vi "blink_if_zero.vi"(8 "error in (no error)":errorcluster, 11 "ImagingModeDL100901FlexTrajectory in":refnum<class "ImagingModeDL100901FlexTrajectory.lvclass">) -> (0 "error out":errorcluster, 3 "ImagingModeDL100901FlexTrajectory out":refnum<class "ImagingModeDL100901FlexTrajectory.lvclass">)   [LabVIEW 2010, in "ImagingModeDL100901FlexTrajectory.lvclass"]
uses:
  ImagingModeDL100901FlexTrajectory.lvclass
  ImagingModeDL100901FlexTrajectory.lvclass/ImagingModeDL100901FlexTrajectory.ctl
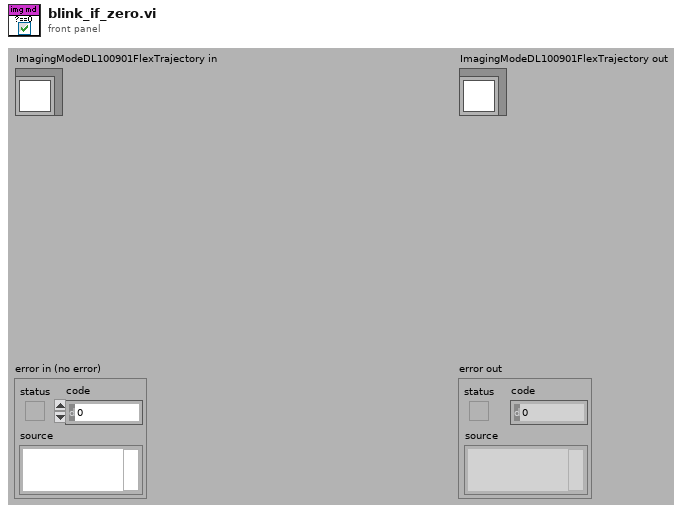
[diagram p1: front panel]
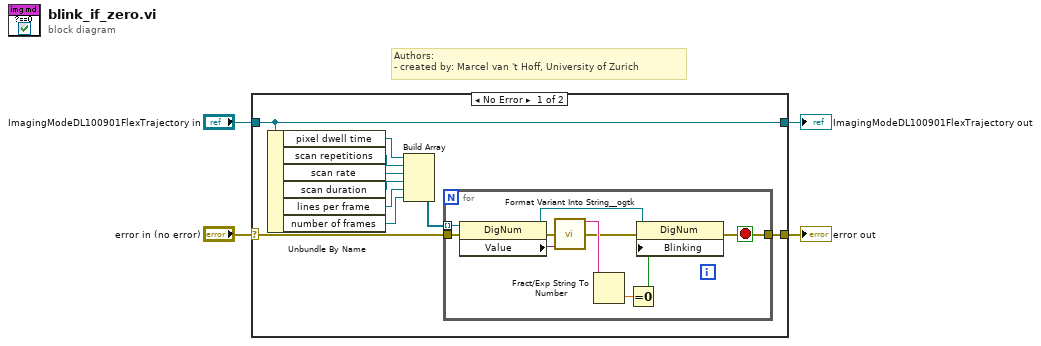
[diagram p0: block diagram]
diagram:
  # "Authors: \n- created by: Marcel van 't Hoff, University of Zurich"
  n1 = case shown="No Error" "error in (no error)" {
    selector: "error in (no error)" -> [w6 w26]
    tunnel: [w5 w26] -> w3
    tunnel: [w14 w25] -> w1
    tunnel: "ImagingModeDL100901FlexTrajectory in" -> [w14 w25]
    frame No Error {
      n2 = Unbundle By Name(w14) -> ("pixel dwell time"=w13:refnum<vi>, "scan repetitions"=w12:refnum<vi>, "scan rate"=w11:refnum<vi>, "scan duration"=w10:refnum<vi>, "lines per frame"=w9:refnum<vi>, "number of frames"=w8:refnum<vi>)
      n3 = Build Array(w13, w12, w11, w10, w9, w8) -> (w7:refnum<vi>[])
      n4 = for {
        tunnel: w7 -> [w24] mode=indexing
        tunnel: w6 -> [w23]
        tunnel: [w22] -> w5
        stop <- w22 stop-if-true
        n5 = property class="DigNum"(reference=w24, error in=w23) -> (reference out=w21:refnum<vi>, error out=w18:errorcluster, "Value"=w19:variant)
        n6 = call <userlib>:"Format Variant Into String__ogtk.vi"("error in (no error)"=w18, "Variant"=w19) -> ("Output String"=w17:string, "error out"=w15:errorcluster)  [unwired: 12 in]
        n7 = Fract/Exp String To Number(string=w17) -> (number=w16:dbl)  [unwired: 3 in, 1 out]
        n8 = Equal To 0?(x=w16) -> (x = 0?=w20:bool)
        n9 = property class="DigNum"(reference=w21, error in=w15, "Blinking"=w20) -> (error out=w22:errorcluster)  [unwired: 1 out]
      }
    }
    frame Error {
    }
  }
  "error out" <- w3
  "ImagingModeDL100901FlexTrajectory out" <- w1
